vi "PXI Clear AO Tasks.vi"(2 "error in":errorcluster) -> (0 "error out":errorcluster)   [LabVIEW 2015]
uses:
  PXI Globals.vi
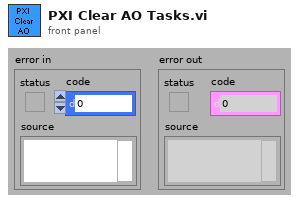
[diagram p1: front panel]
types:
  T1 = typedef "Task Struct.ctl" = cluster{"Task name":string, "Task":refnum<k21>, "Dual-channel task?":bool, "Regenerate?":bool, "Clear?":bool}
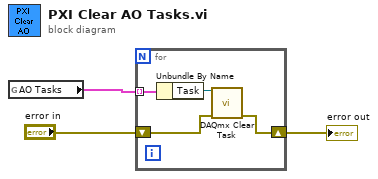
[diagram p0: block diagram]
diagram:
  n1 = global read "PXI Globals.vi" "AO Tasks"() -> (w3:T1[])
  n2 = for {
    tunnel: w3 -> [w7] mode=indexing
    shift-right: [w4] -> w1
    shift-left: "error in" -> [w5]
    n3 = Unbundle By Name(w7) -> ("Task"=w6:refnum<k21>)
    n4 = call <vilib>:"DAQmx Clear Task.vi"("task in"=w6, "error in"=w5) -> ("error out"=w4:errorcluster)  [unwired: 13 in]
  }
  "error out" <- w1
